vi "Query Turret Position (TRIAX).vi"(7 "Mono System # (0)":T2, 8 "error in (no error)":errorcluster, 11 "VISA resource name":refnum<visa-resource-name>) -> (0 "error out":errorcluster, 1 "Groove Density":dbl[unit], 2 "Turret Position":T1, 3 "VISA resource name out":refnum<visa-resource-name>, 4 "Blaze Wavelength":dbl[unit])   [LabVIEW 2023, in "JY-SPEX-TRIAX.lvlib"]
doc: "Queries the turret's position; may be either 0, 1, or 2.\n\n<B>Note: works with TRIAX series spectrometers only.</B>"
uses:
  JY-SPEX-TRIAX.lvlib
  controls.llb/Monochromator System Number.ctl
  controls.llb/Turret Position (TRIAX).ctl
  Spectrometer Config.vi
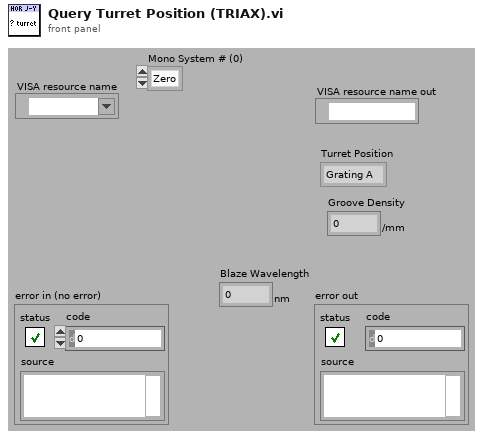
[diagram p1: front panel]
types:
  T1 = typedef "JY-SPEX-TRIAX.lvlib/Turret Position (TRIAX).ctl" = enum16{"Grating A", "Grating B", "Grating C"}
  T2 = typedef "JY-SPEX-TRIAX.lvlib/Monochromator System Number.ctl" = enum16{"Zero", "One"}
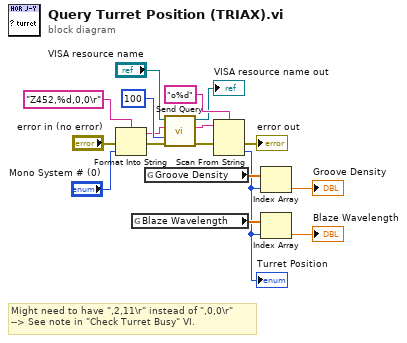
[diagram p0: block diagram]
diagram:
  # "Might need to have \",2,11\\r\" instead of \",0,0\\r\"\n--> See note in \"Check Turret Busy\" VI."
  n1 = Format Into String(format string="Z452,%d,0,0\r", error in="error in (no error)", "Mono System # (0)") -> (resulting string=w13:string, error out=w11:errorcluster)  [unwired: 1 in]
  n2 = global read "Spectrometer Config.vi" "Blaze Wavelength"() -> (w4:dbl[unit][])
  n3 = global read "Spectrometer Config.vi" "Groove Density"() -> (w5:dbl[unit][])
  n4 = call "Send Query.vi"("error in (no error)"=w11, "byte count"=u32 100, "write buffer"=w13, "VISA resource name"="VISA resource name") -> ("error out"=w8:errorcluster, "read buffer"=w10:string, "VISA resource name out"=→"VISA resource name out":refnum<visa-resource-name>)  [unwired: 5 out]
  n5 = Scan From String(format string="o%d", input string=w10, error in=w8) -> (error out=→"error out":errorcluster, output 1=w1:T1)  [unwired: 1 in, 3 out]
  "Turret Position" <- w1
  n6 = Index Array(array=w5, index=w1) -> (element=→"Groove Density":dbl[unit])
  n7 = Index Array(array=w4, index=w1) -> (element=→"Blaze Wavelength":dbl[unit])
